vi "LVIS_GetSAF.vi"(8 "Error In":errorcluster) -> (0 "Error out":errorcluster, 2 "Online?":bool, 3 "SAF State":T1=99 items=["Clear"=0, "SAF Active"=100, "SAF Complete"=101, "SAF > 50%"=102, "SAF < 50%"=103, "SAF Full"=104, "Unknown"=99])   [LabVIEW 2015]
doc: "Polls the Data Commander for the current SAF state value."
uses:
  Ctrls/LVIS_SAF Status.ctl
  Globals/LVIS_DcGlobals.vi
  Globals/LVIS_IsGlobal.vi
panel:
  out "TCP Read":string
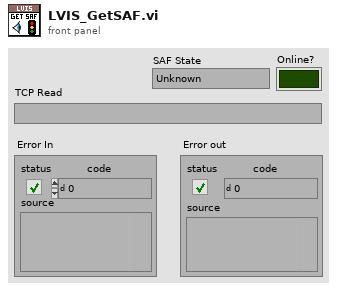
[diagram p1: front panel]
types:
  T1 = typedef "LVIS_SAF Status.ctl" = u16
  T2 = enum16{"Standard", "Buffered", "CRLF", "Immediate"}
  T3 = cluster{"PollRate":string, "ConnTimeout":string, "TxTimeout":string, "RxTimeout":string, "Port":string, "Map":string}
  T4 = cluster{"DCIP":string, "BackupFile":string, "ErrorLog":string, "FilePosition":string}
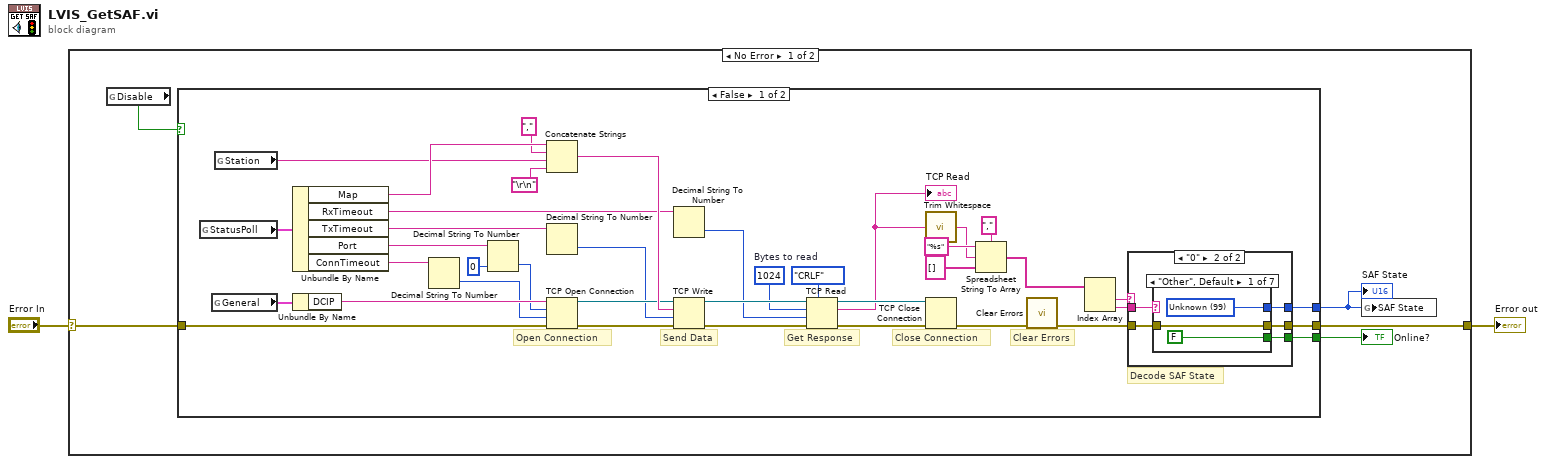
[diagram p0: block diagram]
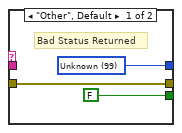
[diagram p2: hidden frame]
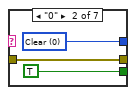
[diagram p3: hidden frame]
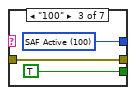
[diagram p4: hidden frame]
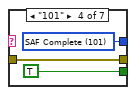
[diagram p5: hidden frame]
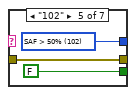
[diagram p6: hidden frame]
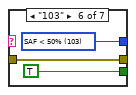
[diagram p7: hidden frame]
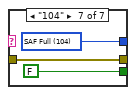
[diagram p8: hidden frame]
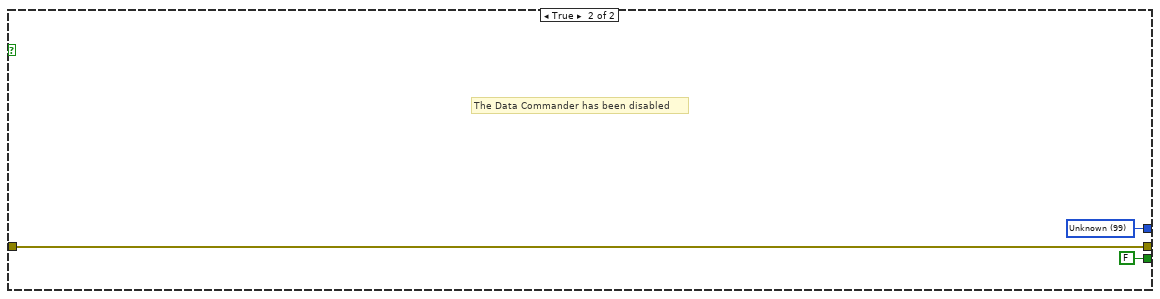
[diagram p9: hidden frame]
diagram:
  n1 = case shown="No Error" "Error In" {
    selector: "Error In" -> [w7 w79]
    tunnel: [w6 w79] -> w1
    frame No Error {
      n2 = global read "LVIS_DcGlobals.vi" "Disable"() -> (w3:bool)
      n3 = case shown="False" w3 {
        tunnel: w7 -> [w36 w78]
        tunnel: [w13 w78] -> w6
        tunnel: [w11 w77] -> w5
        tunnel: [w10 FALSE] -> w4
        frame False {
          w37 = 1024  # Bytes to read
          # "Clear Errors"
          # "Decode SAF State"
          # "Close Connection"
          # "Get Response"
          # "Send Data"
          # "Open Connection"
          n4 = global read "LVIS_DcGlobals.vi" "StatusPoll"() -> (w35:T3)
          n5 = global read "LVIS_DcGlobals.vi" "General"() -> (w34:T4)
          n6 = global read "LVIS_IsGlobal.vi" "Station"() -> (w8:string)
          n7 = Unbundle By Name(w35) -> ("Map"=w24:string, "RxTimeout"=w44:string, "TxTimeout"=w27:string, "Port"=w32:string, "ConnTimeout"=w31:string)
          n8 = Unbundle By Name(w34) -> ("DCIP"=w33:string)
          n9 = Decimal String To Number(string=w31) -> (number=w30:i32)  [unwired: 2 in, 1 out]
          n10 = Decimal String To Number(string=w32, default (0L)=u16 0 ("remote port or service name")) -> (number=w28:u16)  [unwired: 1 in, 1 out]
          n11 = Concatenate Strings(w24, ",", w8, "\r\n") -> (w45:string)
          n12 = Decimal String To Number(string=w27) -> (number=w26:i32)  [unwired: 2 in, 1 out]
          n13 = TCP Open Connection(address=w33, remote port or service name=w28, timeout ms (60000)=w30, error in (no error)=w36) -> (connection ID=w40:refnum<k5>, error out=w39:errorcluster)  [unwired: 1 in]
          n14 = Decimal String To Number(string=w44) -> (number=w25:i32)  [unwired: 2 in, 1 out]
          n15 = TCP Write(connection ID=w40, data in=w45, error in (no error)=w39, 9:w26) -> (connection ID out=w41:refnum<k5>, error out=w46:errorcluster)  [unwired: 1 out]
          n16 = TCP Read(connection ID=w41, bytes to read=w37, error in (no error)=w46, 7:T2."CRLF" ("mode (standard)"), 9:w25) -> (connection ID out=w43:refnum<k5>, data out=w12:string, error out=w42:errorcluster)
          "TCP Read" <- w12
          n17 = call <vilib>:"Trim Whitespace.vi"("string"=w12) -> ("trimmed string"=w17:string)  [unwired: 1 in]
          n18 = TCP Close Connection(connection ID=w43, error in (no error)=w42) -> (error out=w16:errorcluster)  [unwired: 1 in, 1 out]
          n19 = Spreadsheet String To Array(delimiter (Tab)=",", format string="%s", spreadsheet string=w17, array type (2D Dbl)=string[] []) -> (array=w20:string[])
          n20 = call <vilib>:"Clear Errors.vi"("error in (no error)"=w16) -> ("error out"=w9:errorcluster)  [unwired: 5 in, 1 out]
          n21 = Index Array(array=w20) -> (element #1=w15:string, element #2=w14:string)  [unwired: 2 in]
          n22 = case shown="\"0\"" w15 {
            tunnel: w9 -> [w49 w54]
            tunnel: w14 -> [_ w53]
            tunnel: [w49 w52] -> w13
            tunnel: [w48 w51] -> w11
            tunnel: [FALSE w50] -> w10
            frame "Other", Default {
              w48 = T1 99 items=["Clear"=0, "SAF Active"=100, "SAF Complete"=101, "SAF > 50%"=102, "SAF < 50%"=103, "SAF Full"=104, "Unknown"=99] ("SAF Status")
              # "Bad Status Returned"
            }
            frame "0" {
              n23 = case shown="\"Other\", Default" w53 {
                tunnel: w54 -> [w57 w60 w63 w66 w69 w72 w75]
                tunnel: [w57 w60 w63 w66 w69 w72 w75] -> w52
                tunnel: [w56 w59 w62 w65 w68 w71 w74] -> w51
                tunnel: [FALSE TRUE TRUE TRUE FALSE TRUE FALSE] -> w50
                frame "Other", Default {
                  w56 = T1 99 items=["Clear"=0, "SAF Active"=100, "SAF Complete"=101, "SAF > 50%"=102, "SAF < 50%"=103, "SAF Full"=104, "Unknown"=99] ("SAF Status")
                }
                frame "0" {
                  w59 = T1 0 items=["Clear"=0, "SAF Active"=100, "SAF Complete"=101, "SAF > 50%"=102, "SAF < 50%"=103, "SAF Full"=104, "Unknown"=99] ("SAF Status")
                }
                frame "100" {
                  w62 = T1 100 items=["Clear"=0, "SAF Active"=100, "SAF Complete"=101, "SAF > 50%"=102, "SAF < 50%"=103, "SAF Full"=104, "Unknown"=99] ("SAF Status")
                }
                frame "101" {
                  w65 = T1 101 items=["Clear"=0, "SAF Active"=100, "SAF Complete"=101, "SAF > 50%"=102, "SAF < 50%"=103, "SAF Full"=104, "Unknown"=99] ("SAF Status")
                }
                frame "102" {
                  w68 = T1 102 items=["Clear"=0, "SAF Active"=100, "SAF Complete"=101, "SAF > 50%"=102, "SAF < 50%"=103, "SAF Full"=104, "Unknown"=99] ("SAF Status")
                }
                frame "103" {
                  w71 = T1 103 items=["Clear"=0, "SAF Active"=100, "SAF Complete"=101, "SAF > 50%"=102, "SAF < 50%"=103, "SAF Full"=104, "Unknown"=99] ("SAF Status")
                }
                frame "104" {
                  w74 = T1 104 items=["Clear"=0, "SAF Active"=100, "SAF Complete"=101, "SAF > 50%"=102, "SAF < 50%"=103, "SAF Full"=104, "Unknown"=99] ("SAF Status")
                }
              }
            }
          }
        }
        frame True {
          w77 = T1 99 items=["Clear"=0, "SAF Active"=100, "SAF Complete"=101, "SAF > 50%"=102, "SAF < 50%"=103, "SAF Full"=104, "Unknown"=99] ("SAF Status")
          # "The Data Commander has been disabled"
        }
      }
      "SAF State" <- w5
      "Online?" <- w4
      n24 = global write "LVIS_DcGlobals.vi" "SAF State"(w5) -> ()
    }
    frame Error {
    }
  }
  "Error out" <- w1
